vi "4 probe data.vi"() -> ()   [LabVIEW 2014]
doc: "This example shows how to configure multiple channels and acquire waveforms from multiple channels."
uses:
  <vilib>/Analysis/baseanly.llb/Mean (DBL).vi
  <vilib>/MakerHub/LINX/Public/Peripherals/Analog/Analog Read 1 Chan.vi
  <instrlib>/Tektronix TDS 200 1000 2000 Series/Tektronix TDS 200 1000 2000 Series.lvlib
  <vilib>/Analysis/NI_AALBase.lvlib
  <vilib>/MakerHub/LINX/LMH-LINX.lvlib
panel:
  in  "AI Channel 4":u8
  in  "AI Channel 3":u8
  in  "AI Channel 2":u8
  in  "AI Channel 1":u8
  in  "AI Channel 0":u8
  out "Analog Data 0":dbl(graph)
  out "Loop Rate (Hz)":u32
  out "Analog Data 1":dbl(graph)
  out "Analog Data 2":dbl(graph)
  out "Analog Data 3":dbl(graph)
  out "Analog Data 4":dbl(graph)
  out "Numeric":dbl
  in  "Serial Port":refnum<visa-resource-name>
  out "Ch4":dbl
  out "Ch3":dbl
  out "Ch2":dbl
  out "Ch1":dbl
  out "Ch4":waveform(dbl)[](graph)
  out "Ch3":waveform(dbl)[](graph)
  out "Ch2":waveform(dbl)[](graph)
  in  "Channel 4 (3: Channel 4)":u16(ring) items=["Channel 1", "Channel 2", "Channel 3", "Channel 4", "Math", "Reference A", "Reference B", "Reference C", "Reference D"]
  in  "Probe Attenuation 4 (0.1)":dbl=10.0
  in  "Vertical Coupling 4 (1: DC)":u16(ring)=1 items=["AC", "DC", "Ground"]
  in  "Channel 3 (2: Channel 3)":u16(ring) items=["Channel 1", "Channel 2", "Channel 3", "Channel 4", "Math", "Reference A", "Reference B", "Reference C", "Reference D"]
  in  "Probe Attenuation 3 (0.1)":dbl=10.0
  in  "Vertical Coupling 3 (1: DC)":u16(ring)=1 items=["AC", "DC", "Ground"]
  in  "Channel 2 (1: Channel 2)":u16(ring)=1 items=["Channel 1", "Channel 2", "Channel 3", "Channel 4", "Math", "Reference A", "Reference B", "Reference C", "Reference D"]
  in  "Channel 1 (0: Channel 1)":u16(ring) items=["Channel 1", "Channel 2", "Channel 3", "Channel 4", "Math", "Reference A", "Reference B", "Reference C", "Reference D"]
  in  "Serial Configuration":T1={"Baud Rate"=9600, "Parity"=0, "Stop Bits"=10, "Flow Control"=2} {"Flow Control" items=["None", "XON/XOFF", "RTS/CTS", "XON/XOFF & RTS/CTS", "DTR/DSR", "XON/XOFF & DTR/DSR"]; "Stop Bits" items=["1.0"=10, "1.5"=15, "2.0"=20]; "Parity" items=["None", "Odd", "Even", "Mark", "Space"]; "Baud Rate" items=["300"=300, "600"=600, "1200"=1200, "2400"=2400, "4800"=4800, "9600"=9600, "19200"=19200]}
  in  "Probe Attenuation 2 (0.1)":dbl=1.0
  in  "Vertical Coupling 2 (1: DC)":u16(ring)=1 items=["AC", "DC", "Ground"]
  in  "Probe Attenuation 1 (0.1)":dbl=10.0
  in  "Vertical Coupling 1 (1: DC)":u16(ring)=1 items=["AC", "DC", "Ground"]
  in  "Timeout (10000 ms)":u32=10000
  out "Ch1":waveform(dbl)[](graph)
  in  "VISA resource name":refnum<visa-resource-name>
  # "2015 NanoBEEs"
  # "Channel 3"
  # "Channel 1"
  # "Channel 2"
  # "Channel 4"
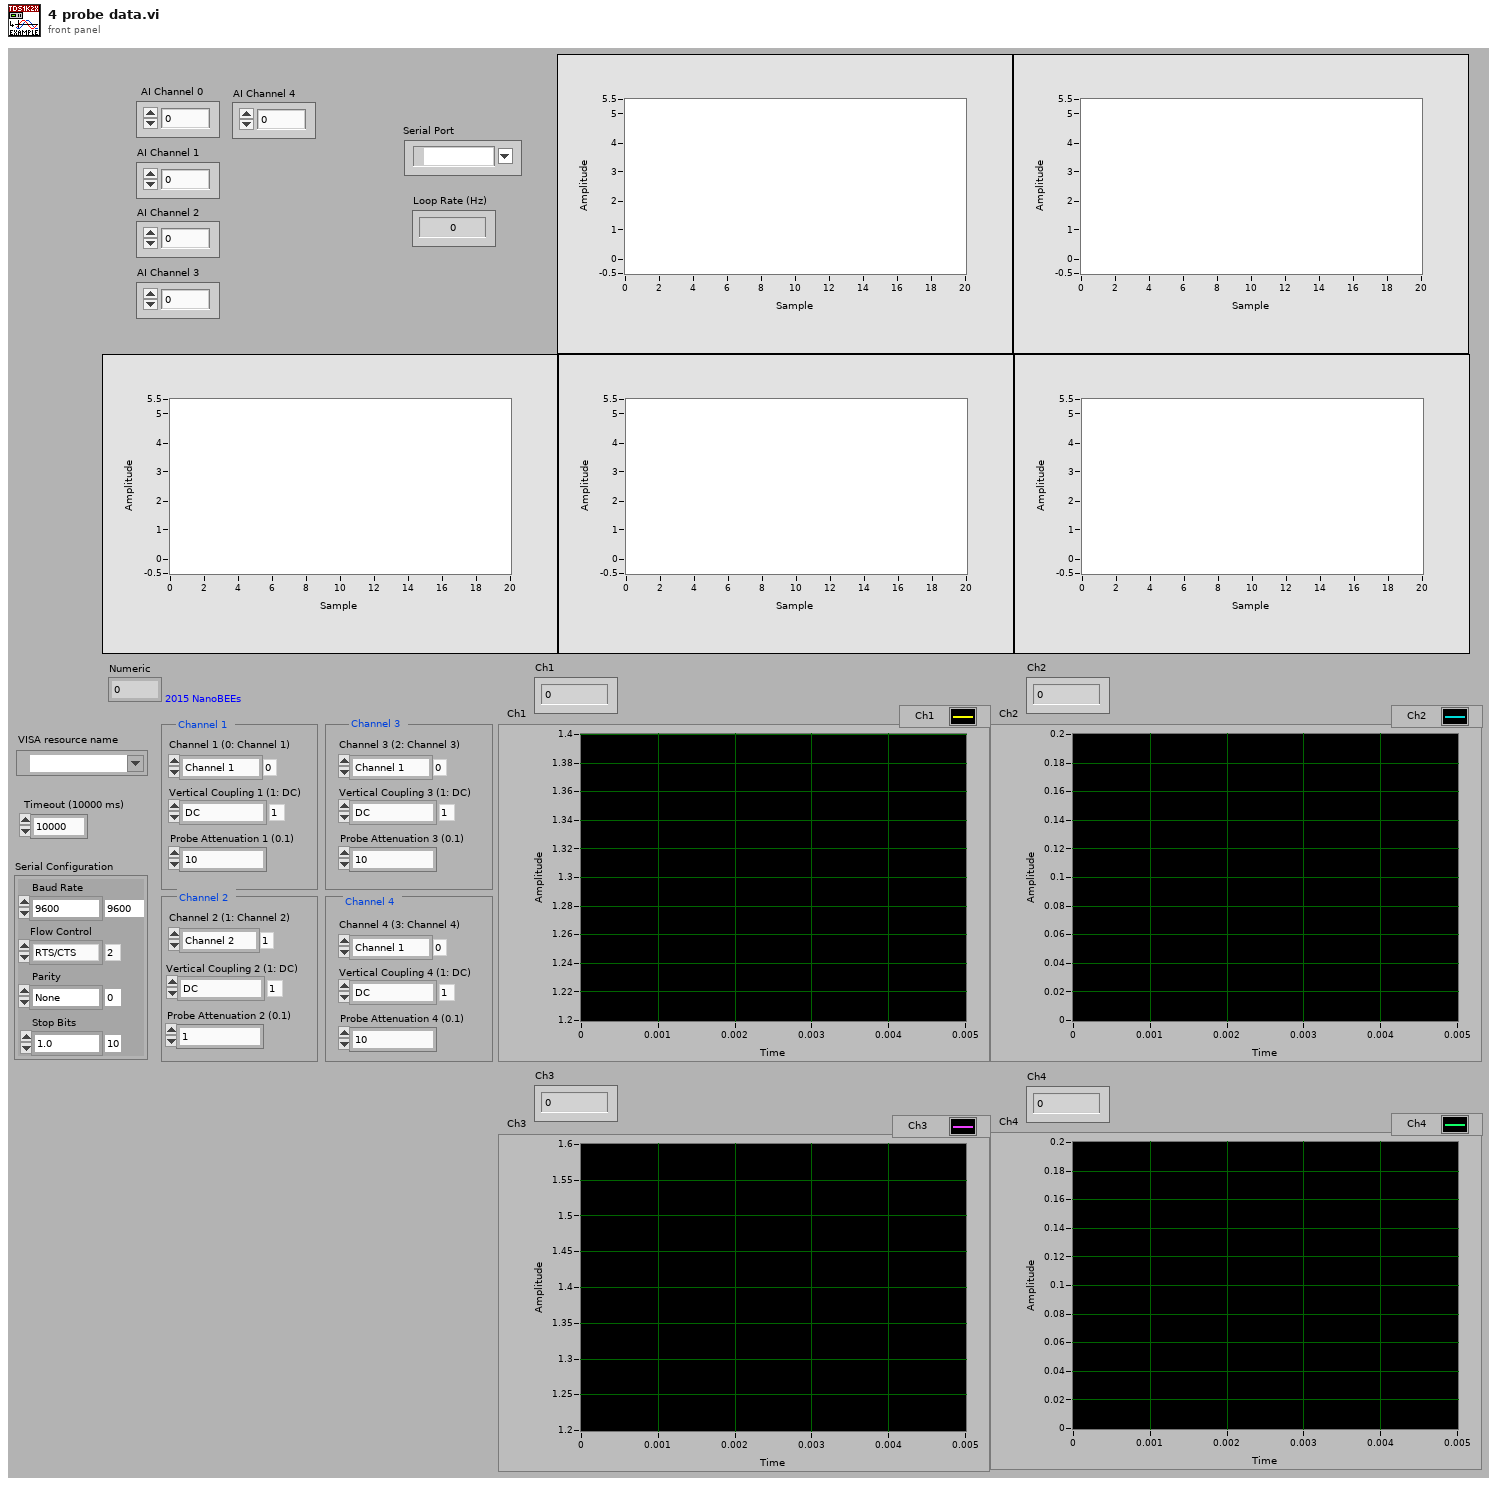
[diagram p1: front panel]
types:
  T1 = cluster{"Baud Rate":u32, "Parity":u16, "Stop Bits":u16, "Flow Control":u16}
  T2 = typedef "LMH-LINX.lvlib/LINX Ref.ctl" = cluster{"Platform":T3, "Interface":T4, "LINX Device Config":T5}
  T3 = typedef "LMH-LINX.lvlib/Platform.ctl" = enum16{"LINX", "myRIO"}
  T4 = typedef "LMH-LINX.lvlib/Interface.ctl" = enum16{"Serial", "TCP"}
  T5 = typedef "LMH-LINX.lvlib/Device.lvlib/LINX Device Config.ctl" = cluster{"Interface":T4, "COM Port":refnum<visa-resource-name>, "TCP Configuration":T6, "Device Family":u8, "Device ID":u8, "Device Name":string, "TCP Ref":refnum<k5>, "Channels":T7}
  T6 = typedef "LMH-LINX.lvlib/Device.lvlib/TCP Config.ctl" = cluster{"IP Address":string, "Port":u16}
  T7 = typedef "LMH-LINX.lvlib/Channels.ctl" = cluster{"DI":u8[], "DO":u8[], "AI":u8[], "AO":u8[], "PWM":u8[], "QE":u8[], "UART":u8[], "I2C 2":u8[], "SPI":u8[], "CAN":u8[], "Servo":u8[], "AI Ref (V)":dbl, "AO Ref (V)":dbl, "AO Resolution (Bits)":u8}
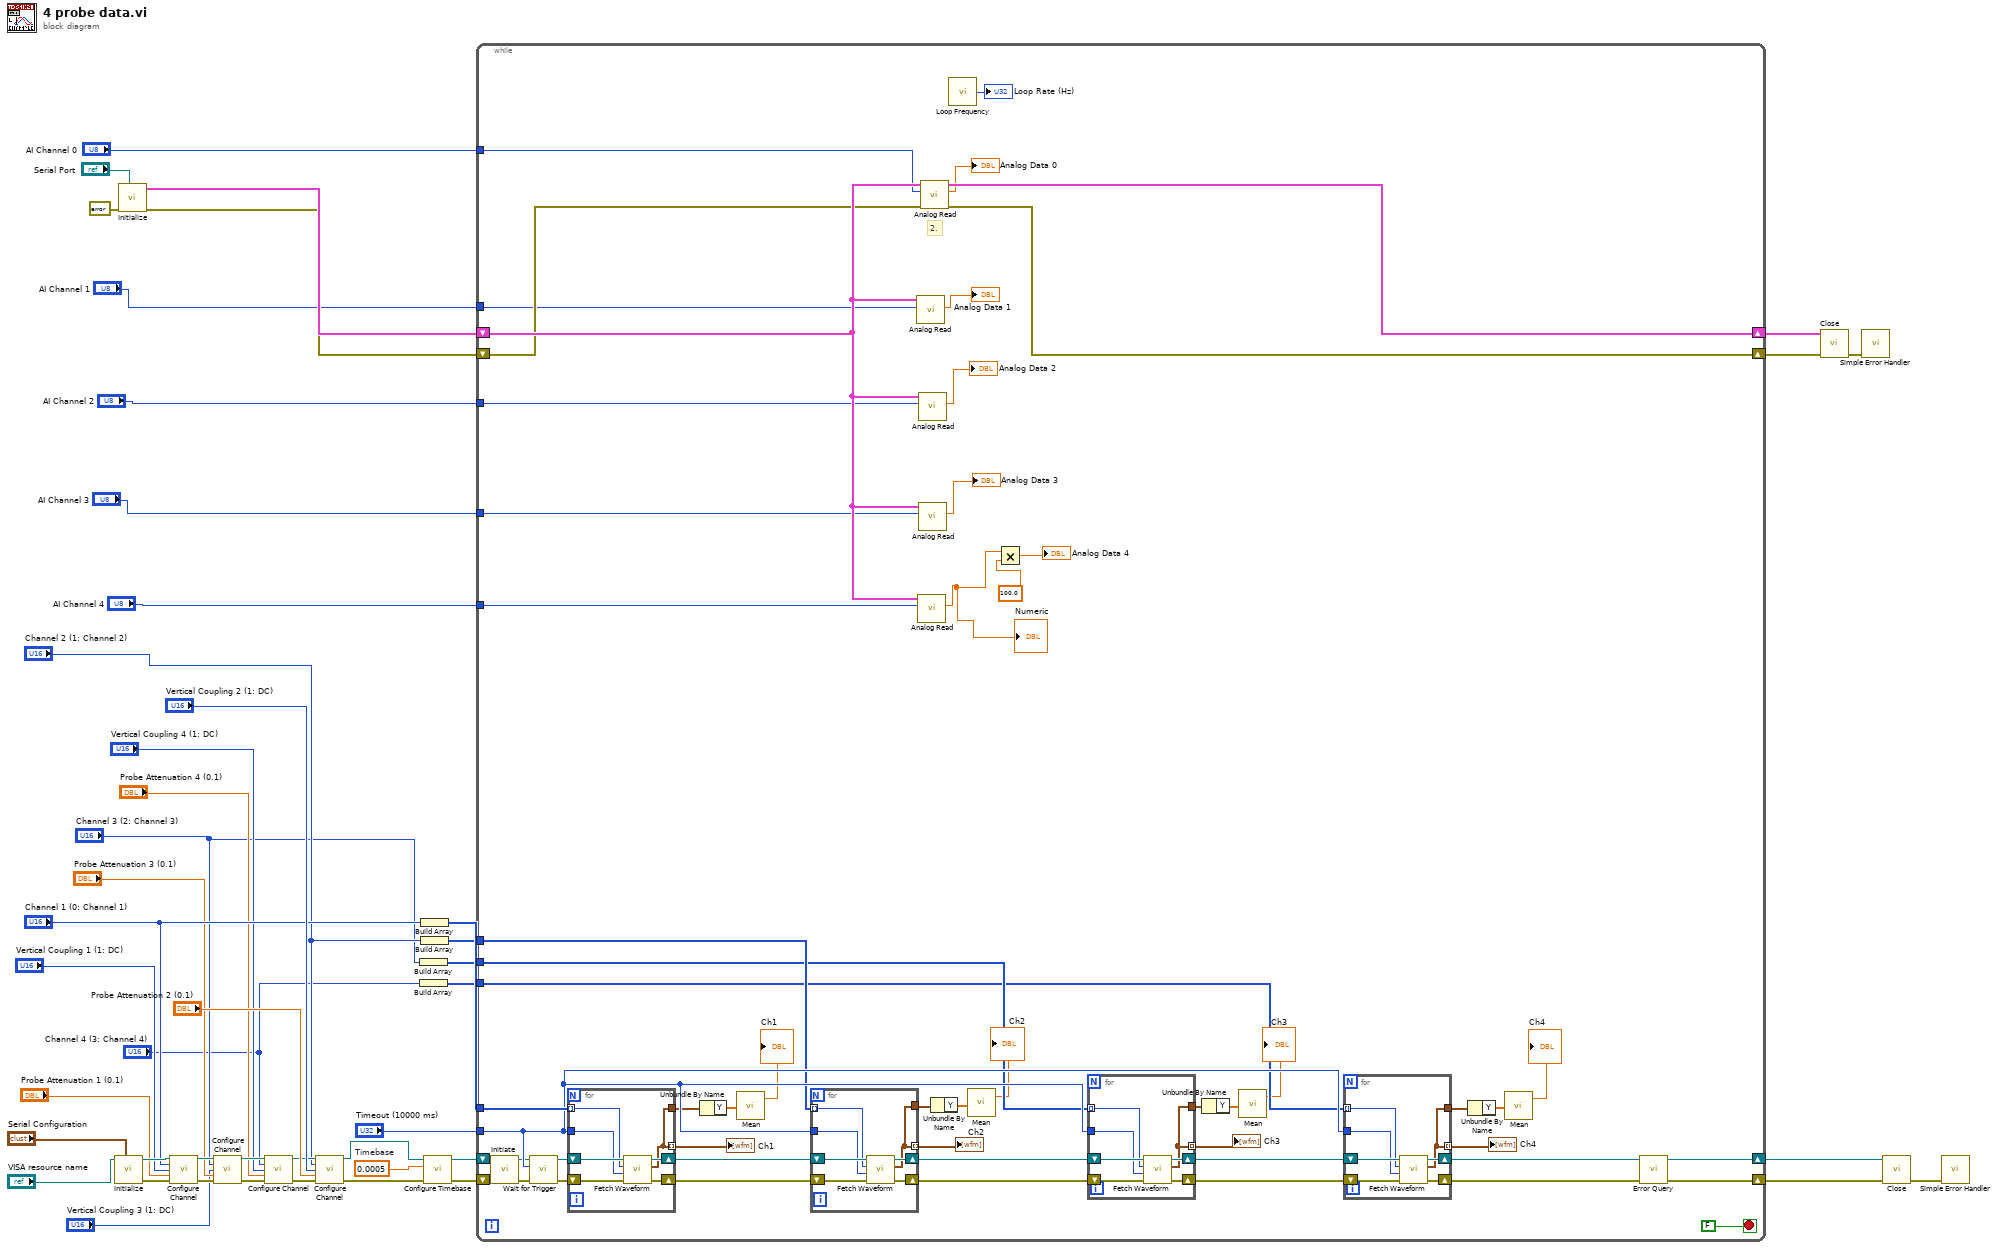
[diagram p0: block diagram]
diagram:
  w33 = 0.0005  # Timebase
  n1 = call <vilib>:"Initialize.vi"("Serial Configuration"="Serial Configuration", "VISA resource name"="VISA resource name") -> ("error out"=w42:errorcluster, "VISA resource name out"=w43:refnum<visa-resource-name>)  [unwired: 3 in, 5 out]
  n2 = call <vilib>:"Initialize.vi"("Serial Port"="Serial Port", "Error In"=errorcluster {"status"=FALSE, "code"=0, "source"=""}) -> ("Error Out"=w11:errorcluster, "LINX Ref"=w12:T2)  [unwired: 7 in, 1 out]
  n3 = call <instrlib>:"Configure Channel.vi"("VISA resource name"=w43, "Channel (0: Channel 1)"="Channel 1 (0: Channel 1)", "Vertical Coupling (1: DC)"="Vertical Coupling 1 (1: DC)", "Probe Attenuation (10: 10X)"="Probe Attenuation 1 (0.1)", "error in (no error)"=w42) -> ("VISA resource name out"=w28:refnum<visa-resource-name>, "error out"=w25:errorcluster)  [unwired: 4 in, 5 out]
  n4 = call <instrlib>:"Configure Channel.vi"("VISA resource name"=w28, "Channel (0: Channel 1)"="Channel 3 (2: Channel 3)", "Vertical Coupling (1: DC)"="Vertical Coupling 3 (1: DC)", "Probe Attenuation (10: 10X)"="Probe Attenuation 3 (0.1)", "error in (no error)"=w25) -> ("VISA resource name out"=w27:refnum<visa-resource-name>, "error out"=w24:errorcluster)  [unwired: 4 in, 5 out]
  n5 = call <instrlib>:"Configure Channel.vi"("VISA resource name"=w27, "Channel (0: Channel 1)"="Channel 4 (3: Channel 4)", "Vertical Coupling (1: DC)"="Vertical Coupling 4 (1: DC)", "Probe Attenuation (10: 10X)"="Probe Attenuation 4 (0.1)", "error in (no error)"=w24) -> ("VISA resource name out"=w26:refnum<visa-resource-name>, "error out"=w23:errorcluster)  [unwired: 4 in, 5 out]
  n6 = call <instrlib>:"Configure Channel.vi"("VISA resource name"=w26, "Channel (0: Channel 1)"="Channel 2 (1: Channel 2)", "Vertical Coupling (1: DC)"="Vertical Coupling 2 (1: DC)", "Probe Attenuation (10: 10X)"="Probe Attenuation 2 (0.1)", "error in (no error)"=w23) -> ("VISA resource name out"=w41:refnum<visa-resource-name>, "error out"=w40:errorcluster)  [unwired: 4 in, 5 out]
  n7 = Build Array("Channel 3 (2: Channel 3)") -> (w14:u16[])
  n8 = Build Array("Channel 4 (3: Channel 4)") -> (w13:u16[])
  n9 = Build Array("Channel 1 (0: Channel 1)") -> (w32:u16[])
  n10 = Build Array("Channel 2 (1: Channel 2)") -> (w17:u16[])
  n11 = call <instrlib>:"Configure Timebase.vi"("error in (no error)"=w40, "Timebase (0.0005 s)"=w33, "VISA resource name"=w41) -> ("error out"=w38:errorcluster, "VISA resource name out"=w39:refnum<visa-resource-name>)  [unwired: 1 in, 6 out]
  n12 = while {
    tunnel: w32 -> [w98]
    tunnel: "Timeout (10000 ms)" -> [w97]
    tunnel: w17 -> [w96]
    tunnel: w14 -> [w95]
    tunnel: w13 -> [w94]
    tunnel: "AI Channel 0" -> [w61]
    tunnel: "AI Channel 1" -> [w60]
    tunnel: "AI Channel 2" -> [w59]
    tunnel: "AI Channel 3" -> [w58]
    tunnel: "AI Channel 4" -> [w57]
    shift-right: [w102] -> w45
    shift-left: w39 -> [w100]
    shift-right: [w101] -> w44
    shift-left: w38 -> [w99]
    shift-right: [w63] -> w10
    shift-left: w12 -> [w65]
    shift-right: [w62] -> w9
    shift-left: w11 -> [w64]
    stop <- FALSE stop-if-true
    # "2."
    n13 = call <instrlib>:"Initiate.vi"("error in (no error)"=w99, "VISA resource name"=w100) -> ("error out"=w90:errorcluster, "VISA resource name out"=w93:refnum<visa-resource-name>)  [unwired: 8 out]
    n14 = call <instrlib>:"Wait for Trigger.vi"("error in (no error)"=w90, "Timeout (10000 ms)"=w97, "VISA resource name"=w93) -> ("error out"=w91:errorcluster, "VISA resource name out"=w92:refnum<visa-resource-name>)  [unwired: 7 out]
    n15 = for {
      shift-right: [w129] -> w87
      shift-left: w91 -> [w127]
      tunnel: w98 -> [w125] mode=indexing
      tunnel: [w124] -> w89 mode=indexing
      tunnel: w97 -> [w126]
      shift-right: [w130] -> w88
      shift-left: w92 -> [w128]
      tunnel: [w124] -> w77
      n16 = call <instrlib>:"Fetch Waveform.vi"("error in (no error)"=w127, "Timeout (10000 ms)"=w126, "Source (0: Channel 1)"=w125, "VISA resource name"=w128) -> ("error out"=w129:errorcluster, "Waveform Data"=w124:waveform(dbl), "VISA resource name out"=w130:refnum<visa-resource-name>)  [unwired: 2 in, 3 out]
    }
    "Ch1" <- w89
    n17 = Unbundle By Name(w77) -> ("Y"=w76:dbl[])
    n18 = call-poly <vilib>:"Mean.vi"("X"=w76) -> ("mean"=→"Ch1":dbl)  [unwired: 1 out]
    n19 = for {
      shift-right: [w122] -> w78
      shift-left: w87 -> [w120]
      tunnel: w96 -> [w118] mode=indexing
      tunnel: [w117] -> w86 mode=indexing
      tunnel: w97 -> [w119]
      shift-right: [w123] -> w79
      shift-left: w88 -> [w121]
      tunnel: [w117] -> w69
      n20 = call <instrlib>:"Fetch Waveform.vi"("error in (no error)"=w120, "Timeout (10000 ms)"=w119, "Source (0: Channel 1)"=w118, "VISA resource name"=w121) -> ("error out"=w122:errorcluster, "Waveform Data"=w117:waveform(dbl), "VISA resource name out"=w123:refnum<visa-resource-name>)  [unwired: 2 in, 3 out]
    }
    "Ch2" <- w86
    n21 = call-poly <vilib>:"Analog Read.vi"("Analog Channel"=w60, "LINX Resource"=w65) -> ("AI Value"=→"Analog Data 1":dbl)  [unwired: 6 in, 3 out]
    n22 = call-poly <vilib>:"Analog Read.vi"("Analog Channel"=w57, "LINX Resource"=w65) -> ("AI Value"=w50:dbl)  [unwired: 6 in, 3 out]
    "Numeric" <- w50
    n23 = call-poly <vilib>:"Analog Read.vi"("Analog Channel"=w59, "LINX Resource"=w65) -> ("AI Value"=→"Analog Data 2":dbl)  [unwired: 6 in, 3 out]
    n24 = call-poly <vilib>:"Analog Read.vi"("Analog Channel"=w58, "LINX Resource"=w65) -> ("AI Value"=→"Analog Data 3":dbl)  [unwired: 6 in, 3 out]
    n25 = call-poly <vilib>:"Analog Read.vi"("Error In"=w64, "Analog Channel"=w61, "LINX Resource"=w65) -> ("Error Out"=w62:errorcluster, "AI Value"=→"Analog Data 0":dbl, "LINX Resource"=w63:T2)  [unwired: 5 in, 1 out]
    n26 = Unbundle By Name(w69) -> ("Y"=w68:dbl[])
    n27 = call <vilib>:"Loop Frequency.vi"() -> ("Loop Rate (Hz)"=→"Loop Rate (Hz)":u32)
    n28 = call-poly <vilib>:"Mean.vi"("X"=w68) -> ("mean"=→"Ch2":dbl)  [unwired: 1 out]
    n29 = Multiply(x=w50, y=100.0) -> (x*y=→"Analog Data 4":dbl)
    n30 = for {
      shift-right: [w115] -> w82
      shift-left: w78 -> [w113]
      tunnel: w95 -> [w111] mode=indexing
      tunnel: [w110] -> w85 mode=indexing
      tunnel: w97 -> [w112]
      shift-right: [w116] -> w83
      shift-left: w79 -> [w114]
      tunnel: [w110] -> w70
      n31 = call <instrlib>:"Fetch Waveform.vi"("error in (no error)"=w113, "Timeout (10000 ms)"=w112, "Source (0: Channel 1)"=w111, "VISA resource name"=w114) -> ("error out"=w115:errorcluster, "Waveform Data"=w110:waveform(dbl), "VISA resource name out"=w116:refnum<visa-resource-name>)  [unwired: 2 in, 3 out]
    }
    "Ch3" <- w85
    n32 = Unbundle By Name(w70) -> ("Y"=w67:dbl[])
    n33 = call-poly <vilib>:"Mean.vi"("X"=w67) -> ("mean"=→"Ch3":dbl)  [unwired: 1 out]
    n34 = for {
      shift-right: [w108] -> w80
      shift-left: w82 -> [w106]
      tunnel: w94 -> [w104] mode=indexing
      tunnel: [w103] -> w84 mode=indexing
      tunnel: w97 -> [w105]
      shift-right: [w109] -> w81
      shift-left: w83 -> [w107]
      tunnel: [w103] -> w71
      n35 = call <instrlib>:"Fetch Waveform.vi"("error in (no error)"=w106, "Timeout (10000 ms)"=w105, "Source (0: Channel 1)"=w104, "VISA resource name"=w107) -> ("error out"=w108:errorcluster, "Waveform Data"=w103:waveform(dbl), "VISA resource name out"=w109:refnum<visa-resource-name>)  [unwired: 2 in, 3 out]
    }
    "Ch4" <- w84
    n36 = Unbundle By Name(w71) -> ("Y"=w66:dbl[])
    n37 = call-poly <vilib>:"Mean.vi"("X"=w66) -> ("mean"=→"Ch4":dbl)  [unwired: 1 out]
    n38 = call <instrlib>:"Error Query.vi"("error in (no error)"=w80, "VISA resource name"=w81) -> ("error out"=w101:errorcluster, "VISA resource name out"=w102:refnum<visa-resource-name>)  [unwired: 8 out]
  }
  n39 = call <instrlib>:"Close.vi"("Error In"=w9, "LINX Resource"=w10) -> ("Error Out"=w7:errorcluster)  [unwired: 8 in, 1 out]
  n40 = call <vilib>:"Simple Error Handler.vi"("error in (no error)"=w7) -> ()  [unwired: 4 in, 5 out]
  n41 = call <instrlib>:"Close.vi"("error in (no error)"=w44, "VISA resource name"=w45) -> ("error out"=w46:errorcluster)  [unwired: 9 out]
  n42 = call <vilib>:"Simple Error Handler.vi"("error in (no error)"=w46) -> ()  [unwired: 1 in, 8 out]
